vi "Save_tracker_settings.vi"(0 "PORT NAME":string="Inlet_Heaters", 1 "Set":enum16{"Set", "Read"}(ring)) -> ()   [LabVIEW 2011]
uses:
  Anemometry/Anemometry Sub Vis/Globals/Constants_global.vi
panel:
  out "Comments":string[](array[string])
  out "Good Reply?":bool[](array[boolean])
  in  "Module Addresses":i32[](array[numeric])=[101, 102, 103, 104, 105, 106, 107, 108, 109, 110, 111, 112, 113, 114, 115]
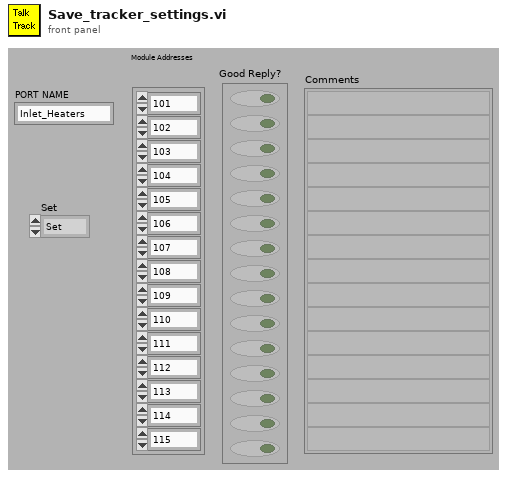
[diagram p1: front panel]
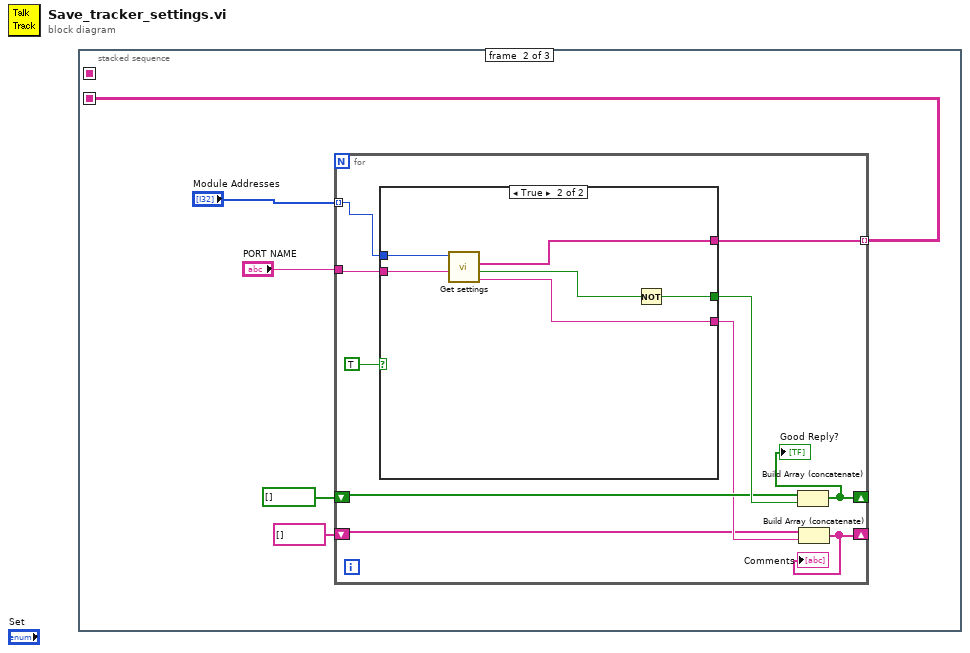
[diagram p0: block diagram]
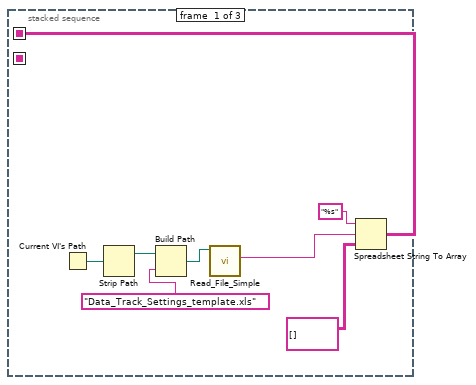
[diagram p2: hidden frame]
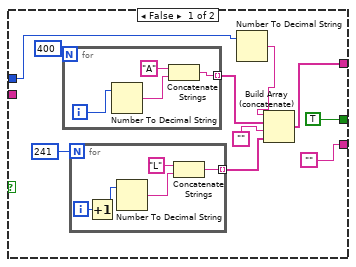
[diagram p3: hidden frame]
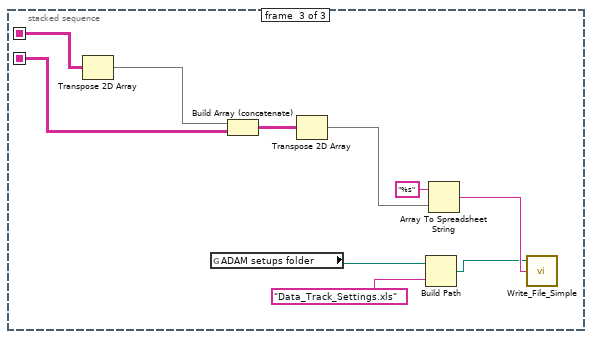
[diagram p4: hidden frame]
diagram:
  n1 = stacked-sequence {
    seq-local: [_ w11 _] -> [_ _ w56]
    seq-local: [w1 _ _] -> [_ _ w58]
    frame #0 {
      n2 = Current VI's Path() -> (path=w8:path)
      n3 = Strip Path(path=w8) -> (stripped path=w7:path)  [unwired: 1 out]
      n4 = Build Path(base path=w7, name or relative path="Data_Track_Settings_template.xls") -> (appended path=w5:path)
      n5 = call "Read_File_Simple.vi"("Filename"=w5) -> ("string"=w4:string)  [unwired: 4 in, 5 out]
      n6 = Spreadsheet String To Array(format string="%s", spreadsheet string=w4, array type (2D Dbl)=string[][] []) -> (array=w1:string[][])  [unwired: 1 in]
    }
    frame #1 {
      n7 = for {
        tunnel: "Module Addresses" -> [w22] mode=indexing
        tunnel: "PORT NAME" -> [w23]
        tunnel: [w21] -> w11 mode=indexing
        shift-right: [w14] -> _
        shift-left: bool[] [] -> [w18]
        shift-right: [w15] -> _
        shift-left: string[] [] -> [w16]
        n8 = case shown="True" TRUE {
          tunnel: w23 -> [_ w48]
          tunnel: w22 -> [w25 w47]
          tunnel: [TRUE ("Error") w43] -> w19
          tunnel: ["" w45] -> w17
          tunnel: [w28 w44] -> w21
          frame False {
            n9 = for {
              N: 400 -> [_]
              tunnel: [w39] -> w31 mode=indexing
              i -> [w42]
              n10 = Number To Decimal String(number=w42) -> (decimal integer string=w41:string)  [unwired: 1 in]
              n11 = Concatenate Strings("A" ("string"), w41) -> (w39:string)
            }
            n12 = for {
              N: 241 -> [_]
              tunnel: [w34] -> w30 mode=indexing
              i -> [w38]
              n13 = Increment(x=w38) -> (x+1=w35:i32)
              n14 = Number To Decimal String(number=w35) -> (decimal integer string=w37:string)  [unwired: 1 in]
              n15 = Concatenate Strings("L" ("string"), w37) -> (w34:string)
            }
            n16 = Number To Decimal String(number=w25) -> (decimal integer string=w24:string)  [unwired: 1 in]
            n17 = Build Array (concatenate)(w24, w31, "", w30) -> (w28:string[])
          }
          frame True {
            n18 = call "Get settings.vi"("MODULE ADDRESS"=w47, "PORT NAME"=w48) -> ("Settings"=w44:string[], "Error"=w46:bool, "Comments"=w45:string)  [unwired: 6 in]
            n19 = Not(x=w46) -> (.not. x?=w43:bool)
          }
        }
        n20 = Build Array (concatenate)(w18, w19) -> (w14:bool[])
        "Good Reply?" <- w14
        n21 = Build Array (concatenate)(w16, w17) -> (w15:string[])
        "Comments" <- w15
      }
    }
    frame #2 {
      n22 = Transpose 2D Array(2D array=w58) -> (transposed array=w57:string[][])
      n23 = global read "Constants_global.vi" "ADAM setups folder"() -> (w51:path)
      n24 = Build Array (concatenate)(w57, w56) -> (w55:string[][])
      n25 = Transpose 2D Array(2D array=w55) -> (transposed array=w54:string[][])
      n26 = Build Path(base path=w51, name or relative path="Data_Track_Settings.xls") -> (appended path=w49:path)
      n27 = Array To Spreadsheet String(array=w54, 3:"%s" ("format string")) -> (spreadsheet string=w52:string)  [unwired: 1 in]
      n28 = call "Write_File_Simple.vi"("character string"=w52, "file path"=w49) -> ()  [unwired: 1 in, 2 out]
    }
  }
